vi "Main.vi"() -> ()   [LabVIEW 2026]
uses:
  01_Data_Types/BTMS_States.ctl
  01_Data_Types/Hardware_State.ctl
  01_Data_Types/Thermal_Logic_Results.ctl
  01_Data_Types/Test_Settings.ctl
  01_Data_Types/BTMS_Main_Data.ctl
panel:
  in  "stop":bool
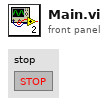
[diagram p1: front panel]
types:
  T1 = typedef "BTMS_Main_Data.ctl" = cluster{"Hardware_State":T2, "Thermal_Logic_Results":T3, "Test_Settings":T4, "System Error":errorcluster, "BTMS_States":T5}
  T2 = typedef "Hardware_State.ctl" = cluster{"Voltage":dbl, "Current":dbl, "Cell_Temperatures":dbl[], "Ambient_Temp":dbl, "Fan_Speed_Actual":i32}
  T3 = typedef "Thermal_Logic_Results.ctl" = cluster{"Heat_Gen_Rate":dbl, "Thermal_Resistance":dbl, "Internal_Resistance":dbl, "Estimated_SoC":dbl}
  T4 = typedef "Test_Settings.ctl" = cluster{"Max_Temp_Limit":dbl, "Cutoff_Voltage":dbl, "Charge_Current_Set":dbl, "Data_Log_Rate":dbl}
  T5 = typedef "BTMS_States.ctl" = enum16{"Initialize", "Idle", "Charging", "Fault", "Exit"}
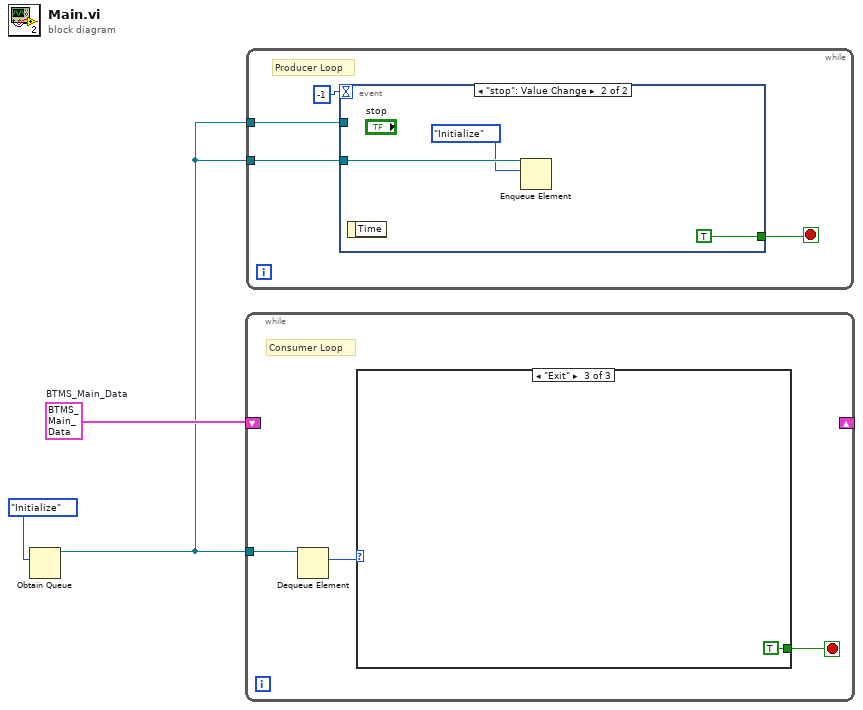
[diagram p0: block diagram]
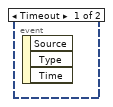
[diagram p2: hidden frame]
diagram:
  w2 = T1 {"Hardware_State"={"Voltage"=0.0, "Current"=0.0, "Cell_Temperatures"=[], "Ambient_Temp"=0.0, "Fan_Speed_Actual"=0}, "Thermal_Logic_Results"={"Heat_Gen_Rate"=0.0, "Thermal_Resistance"=0.0, "Internal_Resistance"=0.0, "Estimated_SoC"=0.0}, "Test_Settings"={"Max_Temp_Limit"=0.0, "Cutoff_Voltage"=0.0, "Charge_Current_Set"=0.0, "Data_Log_Rate"=0.0}, "System Error"={"status"=FALSE, "code"=0, "source"=""}, "BTMS_States"=enum."Idle"}  # BTMS_Main_Data
  n1 = Obtain Queue(element data type=BTMS_States."Initialize" ("BTMS_States")) -> (queue out=w1:refnum<queue>)  [unwired: 4 in, 2 out]
  n2 = while {
    shift-right: _ -> [_]
    shift-left: w2 -> [_]
    tunnel: w1 -> [w6]
    stop <- w4 stop-if-true
    # "Consumer Loop"
    n3 = Dequeue Element(queue=w6) -> (element=w5:T5)  [unwired: 2 in, 3 out]
    n4 = case shown="\"Exit\"" w5 {
      tunnel: [_ _ TRUE] -> w4
      frame "Initialize", Default {
      }
      frame "Idle" {
      }
      frame "Exit" {
      }
    }
  }
  n5 = while {
    tunnel: w1 -> [w10]
    tunnel: w1 -> [w8]
    stop <- w9 stop-if-true
    # "Producer Loop"
    n6 = event shown="[1] \"stop\": Value Change" {
      selector: _ -> [_ _]
      dyn-events: _ -> [_ _]
      timeout: -1 -> [_ _]
      tunnel: w10 -> [_ _]
      tunnel: [_ TRUE] -> w9
      tunnel: w8 -> [_ w13]
      event Timeout {
        n7 = event-data() -> ()  [unwired: 1 in, 3 out]
      }
      event "stop": Value Change {
        n8 = event-data() -> ()  [unwired: 1 in, 1 out]
        n9 = Enqueue Element(queue=w13, element=BTMS_States."Initialize") -> ()  [unwired: 2 in, 3 out]
      }
    }
  }
